vi "Main VI w_o ring implementing Bluetooth.vi"() -> ()   [LabVIEW 2017]
uses:
  data.ctl
  caseControl.ctl
  data cluster.ctl
  <vilib>/Utility/error.llb/DialogType.ctl
  <vilib>/Instr/_visa.llb/VISA Configure Serial Port (Instr).vi
  <vilib>/Analysis/3filter.llb/Butterworth Filter (DBL).vi
  <vilib>/Analysis/NI_AALBase.lvlib
panel:
  out "Input Data":waveform(dbl)(graph)
  out "Filtered Data":dbl[](graph)
  in  "Vibe intensity":u8
  out "Index Volt":string
  out "Thumb Volt":string
  in  "Stop Button":bool
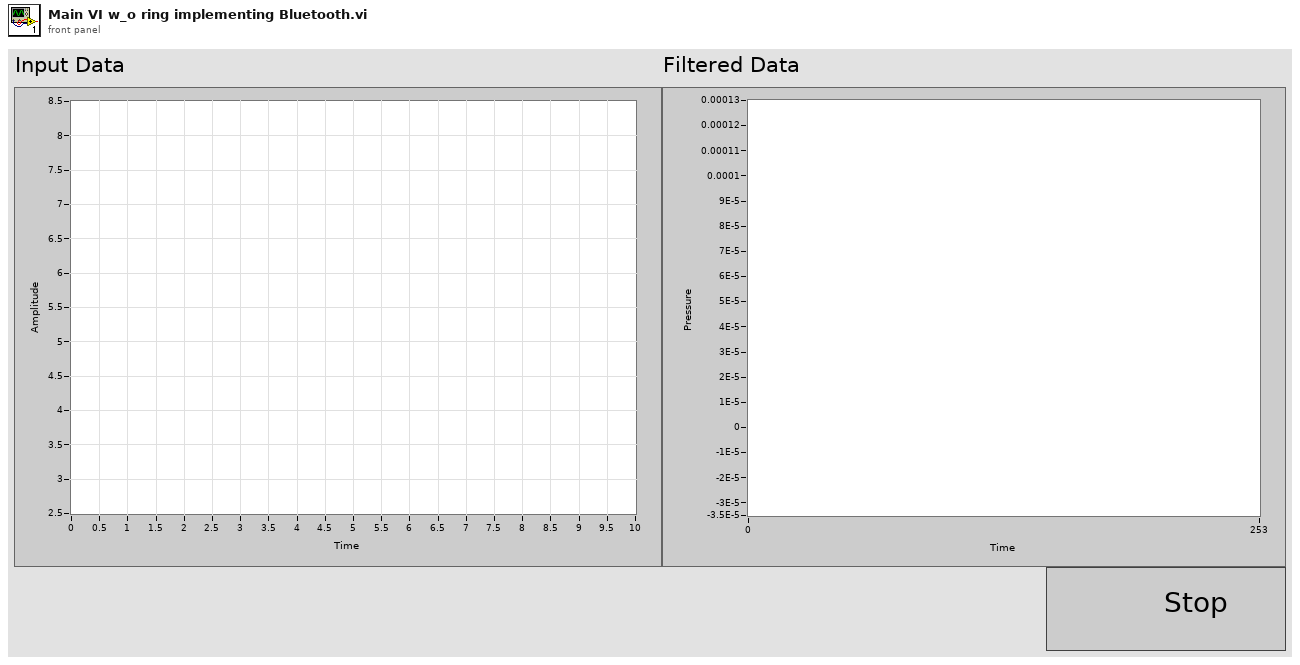
[diagram p1: front panel]
types:
  T1 = typedef "DialogType.ctl" = u16
  T2 = typedef "data cluster.ctl" = cluster{"Pressure":dbl[], "Waveform":waveform(dbl), "Voltage":dbl[]}
  T3 = enum16{"open", "replace", "create", "open or create", "replace or create", "replace or create with confirmation"}
  T4 = typedef "caseControl.ctl" = enum16{"Initialize", "Wait for Event", "Convert Signal", "Noise Processing", "Threshold Processing", "Stop"}
  T5 = typedef "data.ctl" = cluster{"First Name:":string, "Last Name:":string, "Threshold Number:":dbl}
  T6 = cluster{"First Name:":string, "Last Name:":string, "Threshold number:":dbl}
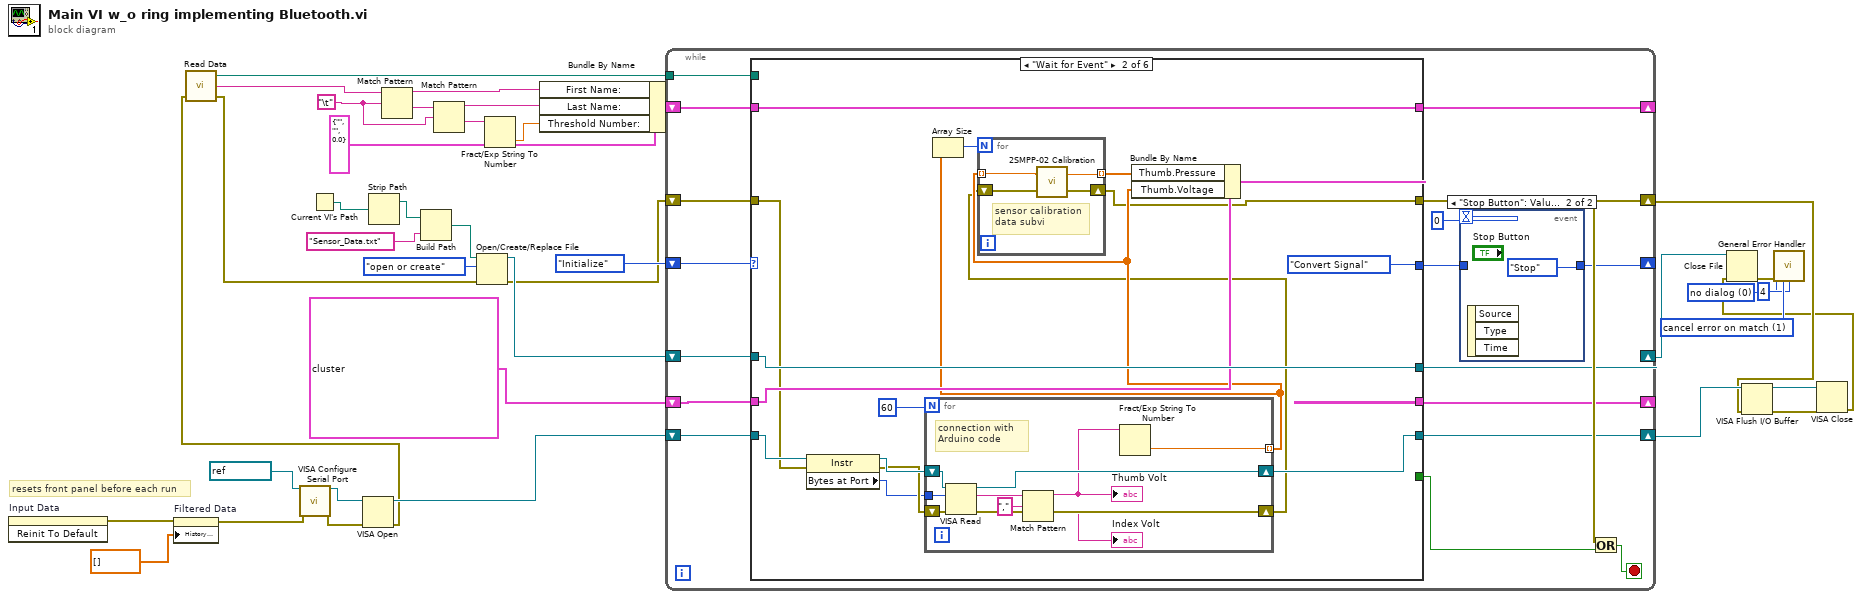
[diagram p0: block diagram]
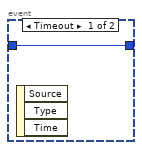
[diagram p2: hidden frame]
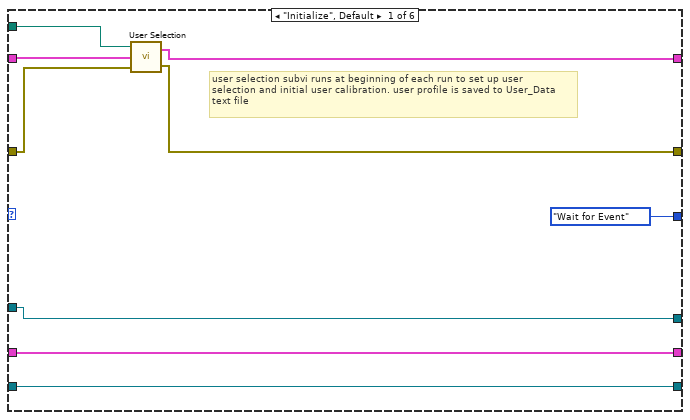
[diagram p3: hidden frame]
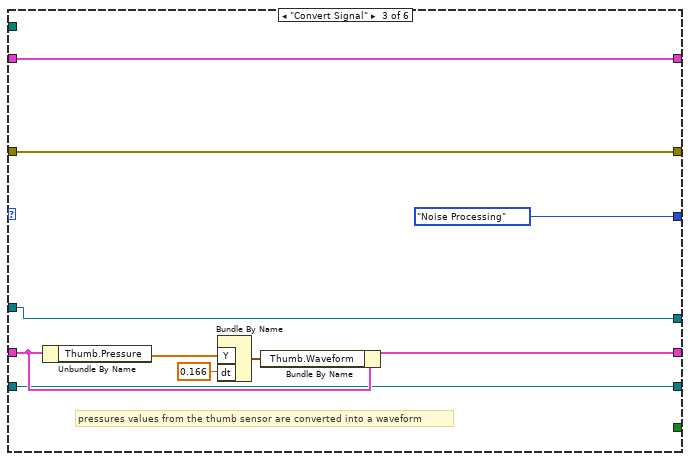
[diagram p4: hidden frame]
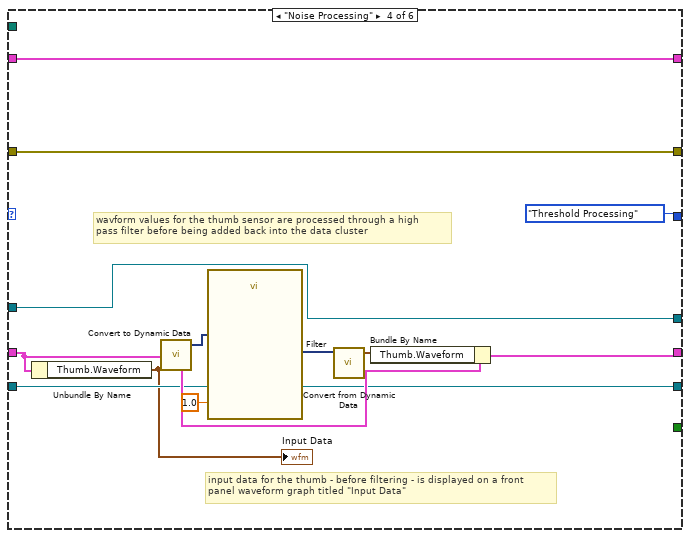
[diagram p5: hidden frame]
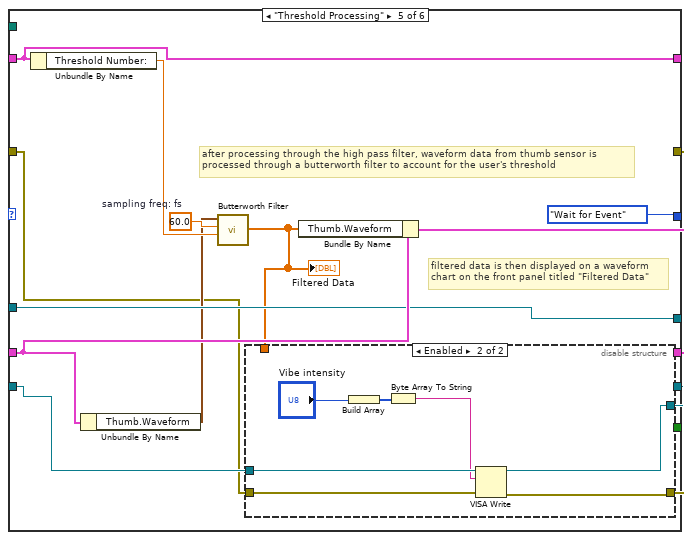
[diagram p6: hidden frame]
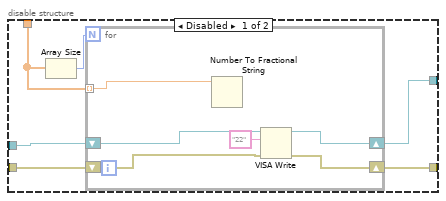
[diagram p7: hidden frame]
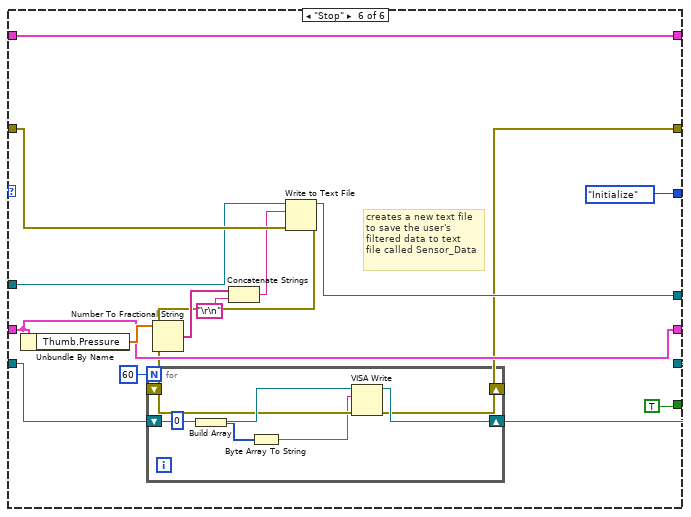
[diagram p8: hidden frame]
diagram:
  w2 = T1 0 items=["no dialog", "OK message", "continue or stop message", "OK message + warnings", "continue/stop + warnings"] ("type of dialog (OK msg:1)")
  w21 = 1 items=["no exception", "cancel error on match", "set error on match"] ("[exception action] (none:0)")
  w37 = "\t"
  # "resets front panel before each run"
  n1 = invoke on="Input Data" class="WFGraph (strict)" method="Reinit To Default"() -> (error out=w1:errorcluster)  [unwired: 3 in, 2 out]
  n2 = property on="Filtered Data" class="WFChart (strict)"(error in=w1, "History Data"=dbl[] []) -> (error out=w9:errorcluster)  [unwired: 1 in, 1 out]
  n3 = call-poly "VISA Configure Serial Port"("VISA resource name"=refnum<visa-resource-name> "COM8", "error in (no error)"=w9) -> ("VISA resource name out"=w13:refnum<visa-resource-name>, "error out"=w14:errorcluster)  [unwired: 12 in]
  n4 = Current VI's Path() -> (path=w19:path)
  n5 = VISA Open(error in (no error)=w14, VISA resource name=w13) -> (VISA resource name=w12:refnum<visa-resource-name>, error out=w11:errorcluster)  [unwired: 3 in]
  n6 = call "Read Data.vi"("Error In"=w11) -> ("error out"=w25:errorcluster, "text"=w34:string, "appended path"=w33:path)  [unwired: 2 in]
  n7 = Strip Path(path=w19) -> (stripped path=w18:path)  [unwired: 1 out]
  n8 = Match Pattern(string=w34, regular expression=w37) -> (before substring=w28:string, after substring=w38:string)  [unwired: 1 in, 2 out]
  n9 = Build Path(base path=w18, name or relative path="Sensor_Data.txt") -> (appended path=w16:path)
  n10 = Match Pattern(string=w38, regular expression=w37) -> (before substring=w29:string, after substring=w36:string)  [unwired: 1 in, 2 out]
  n11 = Open/Create/Replace File(file path (use dialog)=w16, error in=w25, operation (0:open)=T3."open or create") -> (refnum out=w26:refnum<file>, error out=w24:errorcluster)  [unwired: 3 in, 1 out]
  n12 = Fract/Exp String To Number(string=w36) -> (number=w30:dbl)  [unwired: 3 in, 1 out]
  n13 = Bundle By Name(cluster=T5 {"First Name:"="", "Last Name:"="", "Threshold Number:"=0.0}, "First Name:"=w28, "Last Name:"=w29, "Threshold Number:"=w30) -> (w31:T5)
  n14 = while {
    shift-right: [w52] -> _
    shift-left: w31 -> [w54]
    shift-right: [w46] -> _
    shift-left: caseControl."Initialize" -> [w55]
    tunnel: w33 -> [w53]
    shift-right: [w49] -> w4
    shift-left: w24 -> [w40]
    shift-right: [w42] -> w23
    shift-left: w26 -> [w45]
    shift-right: [w43] -> _
    shift-left: cluster{"Thumb":T2, "Index":T2} {"Thumb"={"Pressure"=[], "Waveform"={"t0"=timestamp(0 s since 1904-01-01), "dt"=1.0, "Y"=[]}, "Voltage"=[]}, "Index"={"Pressure"=[], "Waveform"={"t0"=timestamp(0 s since 1904-01-01), "dt"=1.0, "Y"=[]}, "Voltage"=[]}} -> [w44]
    shift-right: [w41] -> w7
    shift-left: w12 -> [w39]
    stop <- w50 stop-if-true
    n15 = case shown="\"Wait for Event\"" w55 {
      tunnel: [_ _ _ _ _ TRUE] -> w51
      tunnel: w54 -> [w66 w81 w106 w117 w126 w166]
      tunnel: w40 -> [w65 w73 w107 w118 w120 w162]
      tunnel: w53 -> [w64 _ _ _ _ _]
      tunnel: [caseControl."Wait for Event" caseControl."Convert Signal" caseControl."Noise Processing" caseControl."Threshold Processing" caseControl."Wait for Event" caseControl."Initialize"] -> w47
      tunnel: [w62 w81 w106 w117 w126 w166] -> w52
      tunnel: [w61 w67 w107 w118 w123 w153] -> w49
      tunnel: w45 -> [w59 w78 w99 w112 w127 w161]
      tunnel: [w60 w79 w100 w111 w128 w157] -> w43
      tunnel: w44 -> [w60 w77 w101 w114 w129 w157]
      tunnel: [w59 w78 w99 w112 w127 w160] -> w42
      tunnel: w39 -> [w58 w75 w98 w110 w121 w156]
      tunnel: [w58 w71 w98 w110 w124 w155] -> w41
      frame "Initialize", Default {
        # "user selection subvi runs at beginning of each run to set up user \nselection and initial user calibration. user profile is saved to User_Data\ntext file"
        n16 = call "User Selection.vi"("error in (no error)"=w65, "Cluster"=w66, "file path (use dialog)"=w64) -> ("error out"=w61:errorcluster, "Cluster 2"=w62:T6)
      }
      frame "Wait for Event" {
        n17 = property class="Instr"(reference=w75, error in=w73) -> (reference out=w76:refnum<visa-resource-name>, error out=w74:errorcluster, "Bytes at Port"=w72:u32)
        n18 = for {
          N: 60 -> [_]
          tunnel: w72 -> [w90]
          shift-right: [w89] -> w71
          shift-left: w76 -> [w92]
          shift-right: [w93] -> w68
          shift-left: w74 -> [w91]
          tunnel: [w84] -> w69 mode=indexing
          # "connection with \nArduino code"
          n19 = VISA Read(VISA resource name=w92, byte count=w90, error in (no error)=w91) -> (VISA resource name out=w89:refnum<visa-resource-name>, read buffer=w88:string, error out=w93:errorcluster)  [unwired: 1 out]
          n20 = Match Pattern(string=w88, regular expression=",") -> (before substring=w87:string, after substring=→"Index Volt":string)  [unwired: 1 in, 2 out]
          "Thumb Volt" <- w87
          n21 = Fract/Exp String To Number(string=w87) -> (number=w84:dbl)  [unwired: 3 in, 1 out]
        }
        n22 = Array Size(array=w69) -> (size(s)=w80:i32)
        n23 = for {
          N: w80 -> [_]
          tunnel: [w96] -> w82 mode=indexing
          tunnel: w69 -> [w97] mode=indexing
          shift-right: [w94] -> w67
          shift-left: w68 -> [w95]
          # "sensor calibration\ndata subvi"
          n24 = call "2SMPP-02 Calibration.vi"("error in (no error)"=w95, "Sensor Voltage"=w97) -> ("error out"=w94:errorcluster, "Pressure"=w96:dbl)
        }
        n25 = Bundle By Name(cluster=w77, "Thumb.Pressure"=w82, "Thumb.Voltage"=w69) -> (w79:cluster{"Thumb":T2, "Index":T2})
      }
      frame "Convert Signal" {
        # "pressures values from the thumb sensor are converted into a waveform"
        n26 = Unbundle By Name(w101) -> ("Thumb.Pressure"=w103:dbl[])
        n27 = Bundle By Name("Y"=w103, "dt"=0.166) -> (w102:waveform(dbl))  [unwired: 1 in]
        n28 = Bundle By Name(cluster=w101, "Thumb.Waveform"=w102) -> (w100:cluster{"Thumb":T2, "Index":T2})
      }
      frame "Noise Processing" {
        # "input data for the thumb - before filtering - is displayed on a front\npanel waveform graph titled \"Input Data\""
        # "wavform values for the thumb sensor are processed through a high\npass filter before being added back into the data cluster"
        n29 = Unbundle By Name(w114) -> ("Thumb.Waveform"=w108:waveform(dbl))
        "Input Data" <- w108
        n30 = call "Convert to Dynamic Data"("Waveform"=w108) -> ("Dynamic Data Type"=w109:dynamicdata)  [unwired: 3 in]
        n31 = call "Filter"("Lower Cut-Off"=1.0, "Signal"=w109) -> ("Filtered Signal"=w115:dynamicdata)  [unwired: 8 in, 1 out]
        n32 = call "Convert from Dynamic Data"("Dynamic Data Type"=w115) -> ("Waveform"=w113:waveform(dbl))  [unwired: 3 in]
        n33 = Bundle By Name(cluster=w114, "Thumb.Waveform"=w113) -> (w111:cluster{"Thumb":T2, "Index":T2})
      }
      frame "Threshold Processing" {
        w130 = 60.0  # sampling freq: fs
        # "filtered data is then displayed on a waveform\nchart on the front panel titled \"Filtered Data\""
        # "after processing through the high pass filter, waveform data from thumb sensor is\nprocessed through a butterworth filter to account for the user's threshold"
        n34 = Unbundle By Name(w126) -> ("Threshold Number:"=w131:dbl)
        n35 = Unbundle By Name(w129) -> ("Thumb.Waveform"=w125:waveform(dbl))
        n36 = call-poly <vilib>:"Butterworth Filter.vi"("high cutoff freq: fh"=w131, "sampling freq: fs"=w130, "X"=w125) -> ("Filtered X"=w122:dbl[])  [unwired: 5 in, 1 out]
        "Filtered Data" <- w122
        n37 = disable-structure shown="Enabled" {
          disable-tunnel: w120 -> [w138 w149]
          disable-tunnel: [w137 w150] -> w124
          disable-tunnel: [w136 w148] -> w123
          disable-tunnel: w122 -> [w135 _]
          disable-tunnel: w121 -> [w133 w151]
          frame Disabled {
            n38 = Array Size(array=w135) -> (size(s)=w134:i32)
            n39 = for {
              N: w134 -> [_]
              tunnel: w135 -> [w144] mode=indexing
              shift-right: [w141] -> w137
              shift-left: w133 -> [w142]
              shift-right: [w140] -> w136
              shift-left: w138 -> [w143]
              n40 = Number To Fractional String(number=w144) -> ()  [unwired: 3 in, 1 out]
              n41 = VISA Write(VISA resource name=w142, write buffer="22", error in (no error)=w143) -> (VISA resource name out=w141:refnum<visa-resource-name>, error out=w140:errorcluster)  [unwired: 1 out]
            }
          }
          frame Enabled {
            n42 = Build Array("Vibe intensity") -> (w147:u8[])
            n43 = Byte Array To String(unsigned byte array=w147) -> (string=w146:string)
            n44 = VISA Write(VISA resource name=w151, write buffer=w146, error in (no error)=w149) -> (VISA resource name out=w150:refnum<visa-resource-name>, error out=w148:errorcluster)  [unwired: 1 out]
          }
        }
        n45 = Bundle By Name(cluster=w129, "Thumb.Waveform"=w122) -> (w128:cluster{"Thumb":T2, "Index":T2})
      }
      frame "Stop" {
        # "creates a new text file\nto save the user's \nfiltered data to text \nfile called Sensor_Data"
        n46 = Unbundle By Name(w157) -> ("Thumb.Pressure"=w164:dbl[])
        n47 = Number To Fractional String(number=w164) -> (F-format string=w163:string[])  [unwired: 3 in]
        n48 = Concatenate Strings(w163, "\r\n") -> (w158:string)
        n49 = Write to Text File(file (use dialog)=w161, text=w158, error in=w162) -> (refnum out=w160:refnum<file>, error out=w154:errorcluster)  [unwired: 1 in, 1 out]
        n50 = for {
          N: 60 -> [_]
          shift-right: [w173] -> w155
          shift-left: w156 -> [w174]
          shift-right: [w171] -> w153
          shift-left: w154 -> [w172]
          n51 = Build Array(u8 0 ("Vibe intensity 2")) -> (w169:u8[])
          n52 = Byte Array To String(unsigned byte array=w169) -> (string=w168:string)
          n53 = VISA Write(VISA resource name=w174, write buffer=w168, error in (no error)=w172) -> (VISA resource name out=w173:refnum<visa-resource-name>, error out=w171:errorcluster)  [unwired: 1 out]
        }
      }
    }
    n54 = event shown="[1] \"Stop Button\": Value Change" {
      selector: _ -> [_ _]
      dyn-events: _ -> [_ _]
      timeout: 0 -> [_ _]
      tunnel: w47 -> [w56 _]
      tunnel: [w56 caseControl."Stop"] -> w46
      event Timeout {
        n55 = event-data() -> ()  [unwired: 1 in, 3 out]
      }
      event "Stop Button": Value Change {
        n56 = event-data() -> ()  [unwired: 1 in, 3 out]
      }
    }
    n57 = Or(x=w49, y=w51) -> (x .or. y?=w50:bool)
  }
  n58 = VISA Flush I/O Buffer(VISA resource name=w7, error in (no error)=w4) -> (VISA resource name out=w5:refnum<visa-resource-name>, error out=w6:errorcluster)  [unwired: 1 in]
  n59 = VISA Close(VISA resource name=w5, error in (no error)=w6) -> (error out=w3:errorcluster)
  n60 = Close File(refnum=w23, error in=w3) -> (error out=w22:errorcluster)  [unwired: 1 out]
  n61 = call <vilib>:"General Error Handler.vi"("type of dialog (OK msg:1)"=w2, "error in (no error)"=w22, "[exception action] (none:0)"=w21, "[exception code]"=4) -> ()  [unwired: 7 in, 5 out]
